vi "Off.vi"(8 "error in (no error)":errorcluster, 11 "Lamp in":refnum<class "Lamp.lvclass">) -> (0 "error out":errorcluster, 3 "Lamp out":refnum<class "Lamp.lvclass">)   [LabVIEW 2016, in "Lamp.lvclass"]
uses:
  Lamp.lvclass
  Lamp.lvclass/Lamp.ctl
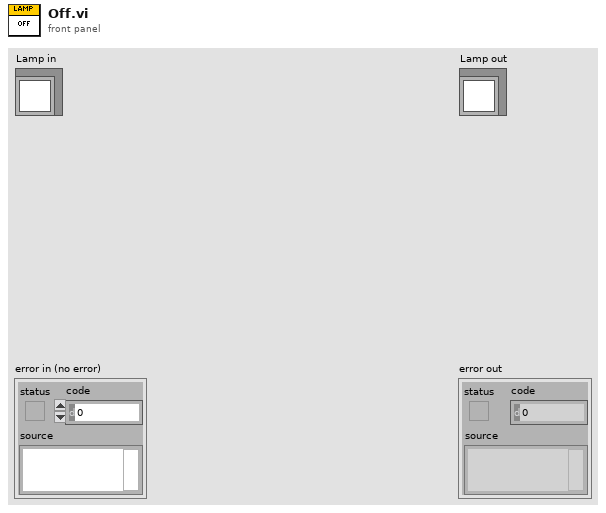
[diagram p1: front panel]
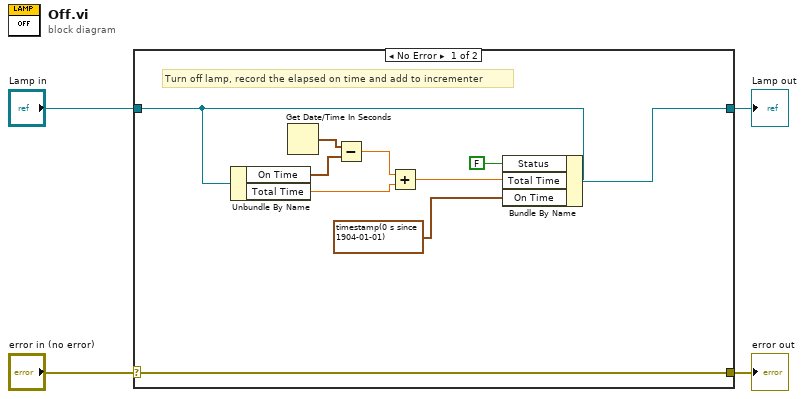
[diagram p0: block diagram]
diagram:
  n1 = case shown="No Error" "error in (no error)" {
    selector: "error in (no error)" -> [w14 w16]
    tunnel: [w14 w16] -> w3
    tunnel: [w13 w15] -> w1
    tunnel: "Lamp in" -> [w12 w15]
    frame No Error {
      # "Turn off lamp, record the elapsed on time and add to incrementer"
      n2 = Unbundle By Name(w12) -> ("On Time"=w9:timestamp, "Total Time"=w7:dbl)
      n3 = Get Date/Time In Seconds() -> (seconds since 1Jan1904=w10:timestamp)
      n4 = Subtract(x=w10, y=w9) -> (x-y=w8:dbl)
      n5 = Add(x=w8, y=w7) -> (x+y=w6:dbl)
      n6 = Bundle By Name(cluster=w12, "Status"=FALSE, "Total Time"=w6, "On Time"=timestamp(0 s since 1904-01-01)) -> (w13:refnum<class "Lamp.lvclass">)
    }
    frame Error {
    }
  }
  "error out" <- w3
  "Lamp out" <- w1
